vi "Global - Pressure & Flow.vi"() -> ()   [LabVIEW 2018]
panel:
  out "Task3 Temperature":dbl=2.13326012312
  out "Task3 Flow Main":dbl=-0.003
  out "Task3 Pressure":dbl=33.89
  out "Task3 Flow Separator":dbl=-0.0039
  in  "Task3 Cycles":i32=100000
  in  "Task3 Ping":bool
  in  "Task3 OK Button":bool
  out "Task3 Time Stamp":timestamp=timestamp(3561050227.07725 s since 1904-01-01)
  out "Task3 error out":errorcluster
  in  "Task3 Stop":bool
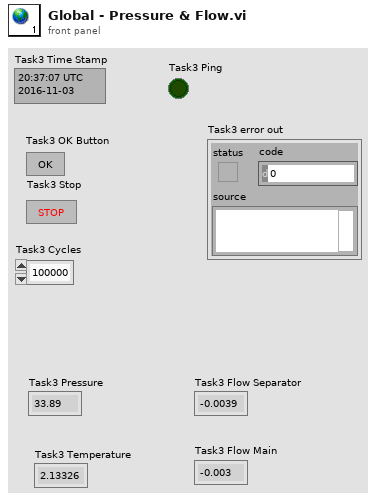
[diagram p1: front panel]
diagram:
